vi "URAPI_SetPWM_num.vi"(0 "Variable In":u8, 3 "URAPI Script":T1={"Script"="", "Whiles"=[], "Ifs"=[], "Supress Err"=TRUE, "Errors"=""}, 4 "Port":u8) -> (2 "Variable Out":string, 5 "URAPI Script":T1={"Script"="", "Whiles"=[], "Ifs"=[], "Supress Err"=TRUE, "Errors"=""})   [LabVIEW 2012]
doc: "Creates a PWM output through the specified \"Port\" according to the specified value of \"Variable in\"."
uses:
  <userlib>/BotSpeak/VIs/Direct/URAPI_Control.ctl
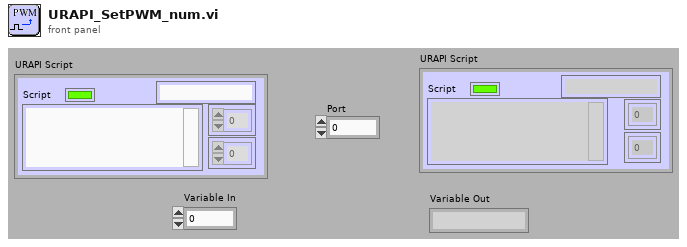
[diagram p1: front panel]
types:
  T1 = typedef "URAPI_Control.ctl" = cluster{"Script":string, "Whiles":u8[], "Ifs":u8[], "Supress Err":bool, "Errors":string}
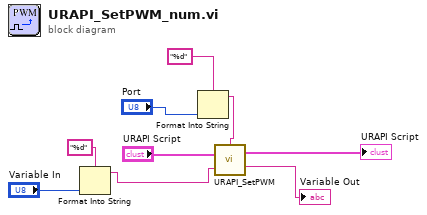
[diagram p0: block diagram]
diagram:
  n1 = Format Into String(format string="%d" ("string"), "Variable In") -> (resulting string=w5:string)  [unwired: 2 in, 1 out]
  n2 = Format Into String(format string="%d" ("string"), "Port") -> (resulting string=w2:string)  [unwired: 2 in, 1 out]
  n3 = call <userlib>:"URAPI_SetPWM.vi"("Variable In"=w5, "URAPI Script"="URAPI Script", "Port"=w2) -> ("Variable Out"=→"Variable Out":string, "URAPI Script"=→"URAPI Script":T1)  [unwired: 1 in]
